vi "Generate Acquisition Parameters.vi"(8 "Error In":errorcluster, 9 "Auto Triggered?":bool, 10 "wfm info":T2(array[cluster])) -> (0 "Error Out":errorcluster, 1 "Acquisition Result":T1={"Traces"=[], "Relative t0 [s]"=1000.0, "Sample Rate [1/s]"=1000.0, "No. of points"=0, "Absolute t0 [s]"=1000.0, "dT [s]"=1000.0, "Update rate [1/s]"=0.0, "Auto Triggered"=FALSE, "Stop"=FALSE} {"Update rate [1/s]" format="%_3p"})   [LabVIEW 2019]
uses:
  Controls/Acquisition Result.ctl
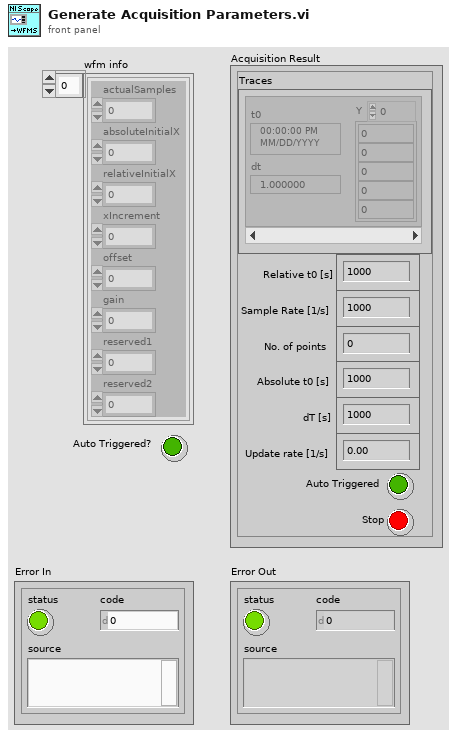
[diagram p1: front panel]
types:
  T1 = typedef "Acquisition Result.ctl" = cluster{"Traces":waveform(sgl)[], "Relative t0 [s]":dbl, "Sample Rate [1/s]":dbl, "No. of points":i32, "Absolute t0 [s]":dbl, "dT [s]":dbl, "Update rate [1/s]":dbl, "Auto Triggered":bool, "Stop":bool}
  T2 = cluster{"actualSamples":i32, "absoluteInitialX":dbl, "relativeInitialX":dbl, "xIncrement":dbl, "offset":dbl, "gain":dbl, "reserved1":dbl, "reserved2":dbl}[]
  T3 = cluster{"actualSamples":i32, "absoluteInitialX":dbl, "relativeInitialX":dbl, "xIncrement":dbl, "offset":dbl, "gain":dbl, "reserved1":dbl, "reserved2":dbl}
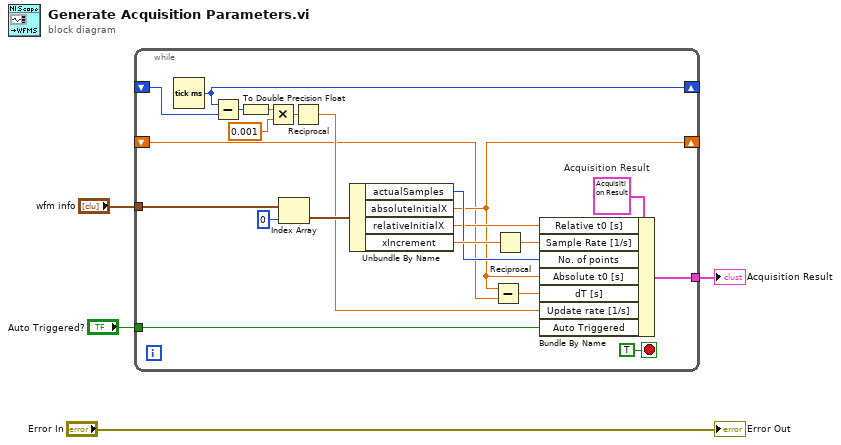
[diagram p0: block diagram]
diagram:
  n1 = while {
    tunnel: "wfm info" -> [w23]
    tunnel: [w11] -> w3
    tunnel: "Auto Triggered?" -> [w10]
    shift-right: [w18] -> _
    shift-left: _ -> [w16]
    shift-right: [w8] -> _
    shift-left: _ -> [w7]
    stop <- TRUE stop-if-true
    w15 = T1 {"Traces"=[], "Relative t0 [s]"=1000.0, "Sample Rate [1/s]"=1000.0, "No. of points"=0, "Absolute t0 [s]"=1000.0, "dT [s]"=1000.0, "Update rate [1/s]"=0.0, "Auto Triggered"=FALSE, "Stop"=FALSE}  # Acquisition Result
    n2 = Tick Count (ms)() -> (millisecond timer value=w18:u32)
    n3 = Subtract(x=w18, y=w16) -> (x-y=w19:u32)
    n4 = To Double Precision Float(number=w19) -> (double precision float=w20:dbl)
    n5 = Multiply(x=w20, y=0.001) -> (x*y=w22:dbl)
    n6 = Index Array(array=w23, index=0) -> (element=w25:T3)
    n7 = Reciprocal(x=w22) -> (1/x=w12:dbl)
    n8 = Unbundle By Name(w25) -> ("actualSamples"=w13:i32, "absoluteInitialX"=w8:dbl, "relativeInitialX"=w9:dbl, "xIncrement"=w14:dbl)
    n9 = Subtract(x=w8, y=w7) -> (x-y=w6:dbl)
    n10 = Reciprocal(x=w14) -> (1/x=w5:dbl)
    n11 = Bundle By Name(cluster=w15, "Relative t0 [s]"=w9, "Sample Rate [1/s]"=w5, "No. of points"=w13, "Absolute t0 [s]"=w8, "dT [s]"=w6, "Update rate [1/s]"=w12, "Auto Triggered"=w10) -> (w11:T1)
  }
  "Acquisition Result" <- w3
  "Error Out" <- "Error In"
